vi "Initialize.vi"(8 "Error in (no error)":errorcluster, 9 "Reset":bool=TRUE caption="Reset (T)", 10 "ID Query":bool=TRUE caption="ID Query (T)", 11 "VISA resource":refnum<visa-resource-name>) -> (0 "Error out":errorcluster, 1 "THM1176 Description":string, 2 "THM1176":bool, 3 "Dup VISA resource":refnum<visa-resource-name>, 4 "Divisors":dbl[](array[numeric]) format="%#_8g", 5 "Ranges":string[](array[string]), 6 "Units":string[](array[string]))   [LabVIEW 2010]
doc: "Copyright (c) 2012 Metrolab Technology SA, Plan-les-Ouates, Geneva, Switzerland\nInitialize the THM1176 LabVIEW API."
panel:
  # "Initialize"
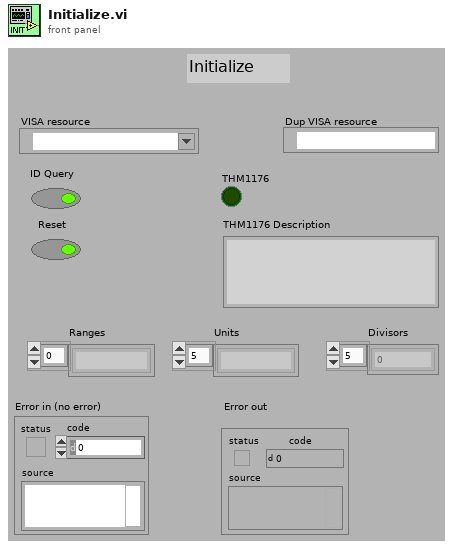
[diagram p1: front panel]
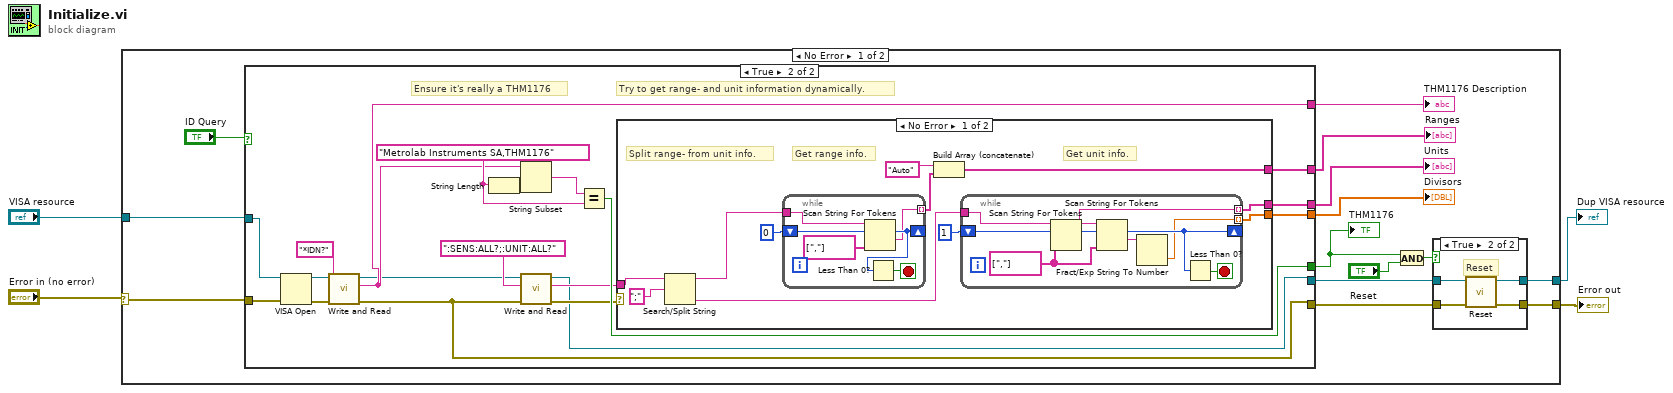
[diagram p0: block diagram]
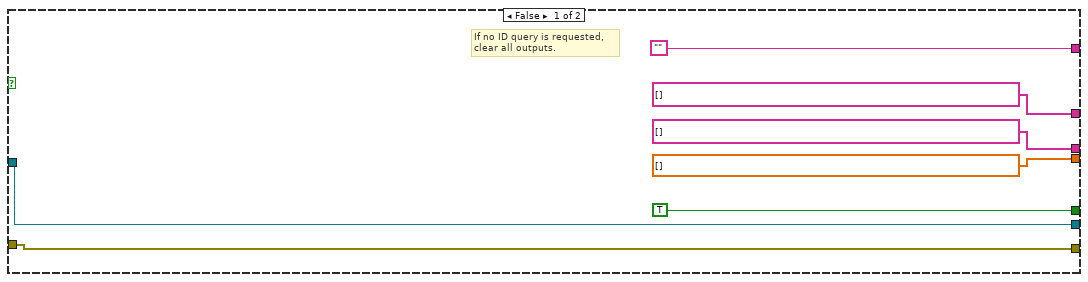
[diagram p2: hidden frame]
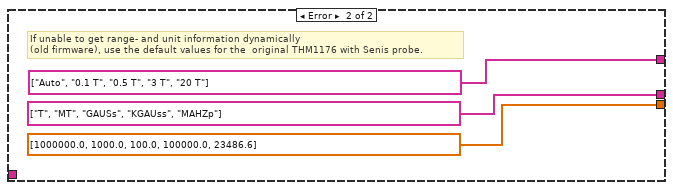
[diagram p3: hidden frame]
diagram:
  n1 = case shown="No Error" "Error in (no error)" {
    selector: "Error in (no error)" -> [w6 w82]
    tunnel: [w15 w81] -> w1
    tunnel: [w14 w82] -> w4
    tunnel: "VISA resource" -> [w5 w81]
    frame No Error {
      n2 = case shown="True" "ID Query" {
        tunnel: w6 -> [w25 w29]
        tunnel: [TRUE w36] -> w11
        tunnel: [w19 w31] -> w18
        tunnel: [w25 w33] -> w17
        tunnel: ["" ("response") w40] -> w13
        tunnel: [string[] [] w39] -> w9
        tunnel: [string[] [] w38] -> w8
        tunnel: [dbl[] [] w37] -> w7
        tunnel: w5 -> [w19 w27]
        frame False {
          # "If no ID query is requested,\nclear all outputs."
        }
        frame True {
          w42 = "Metrolab Instruments SA,THM1176"
          # "Try to get range- and unit information dynamically."
          # "Ensure it's really a THM1176"
          n3 = VISA Open(error in (no error)=w29, VISA resource name=w27) -> (VISA resource name=w26:refnum<visa-resource-name>, error out=w28:errorcluster)  [unwired: 3 in]
          n4 = call "Write and Read.vi"("Error in (no error)"=w28, "Command"="*IDN?" ("string to write"), "VISA resource"=w26) -> ("Error out"=w33:errorcluster, "Response"=w40:string, "Dup VISA resource"=w30:refnum<visa-resource-name>)  [unwired: 4 in, 2 out]
          n5 = String Length(string=w42) -> (length=w43:i32)
          n6 = String Subset(string=w40, length (rest)=w43) -> (substring=w41:string)  [unwired: 1 out]
          n7 = call "Write and Read.vi"("Error in (no error)"=w33, "Command"=":SENS:ALL?;:UNIT:ALL?", "VISA resource"=w30) -> ("Error out"=w34:errorcluster, "Response"=w32:string, "Dup VISA resource"=w31:refnum<visa-resource-name>)  [unwired: 4 in, 2 out]
          n8 = Equal?(x=w41, y=w42) -> (x = y?=w36:bool)
          n9 = case shown="No Error" w34 {
            tunnel: [w46 string[] ["Auto", "0.1 T", "0.5 T", "3 T", "20 T"]] -> w39
            tunnel: [w48 string[] ["T", "MT", "GAUSs", "KGAUss", "MAHZp"]] -> w38
            tunnel: [w47 dbl[] [1000000.0, 1000.0, 100.0, 100000.0, 23486.6]] -> w37
            tunnel: w32 -> [w54 _]
            frame No Error {
              # "Get unit info."
              # "Get range info."
              # "Split range- from unit info."
              n10 = Search/Split String(string=w54, search string/char (-)=";") -> (substring before match=w52:string, match + rest of string=w51:string)  [unwired: 2 out]
              n11 = while {
                shift-right: [w68] -> _
                shift-left: 0 ("offset past token") -> [w71]
                tunnel: w52 -> [w70]
                tunnel: [w66] -> w49 mode=indexing
                stop <- w67 stop-if-true
                n12 = Scan String For Tokens(6:string[] [","] ("delimiters (\\s,\\t,\\r,\\n)"), 8:w71, 9:w70) -> (1:w66:string, 2:w68:i32)  [unwired: 5 out]
                n13 = Less Than 0?(x=w68) -> (x < 0?=w67:bool)
              }
              n14 = Build Array (concatenate)("Auto", w49) -> (w46:string[])
              n15 = while {
                shift-right: [w60] -> _
                shift-left: 1 ("offset past token") -> [w65]
                tunnel: w51 -> [w64]
                tunnel: [w63] -> w48 mode=indexing
                tunnel: [w58] -> w47 mode=indexing
                stop <- w57 stop-if-true
                w61 = string[] [","] ("delimiters (\\s,\\t,\\r,\\n)")
                n16 = Scan String For Tokens(6:w61, 8:w65, 9:w64) -> (1:w63:string, 2:w62:i32, 3:w56:string)  [unwired: 4 out]
                n17 = Scan String For Tokens(6:w61, 8:w62, 9:w56) -> (1:w59:string, 2:w60:i32)  [unwired: 5 out]
                n18 = Fract/Exp String To Number(string=w59) -> (number=w58:dbl)  [unwired: 4 out]
                n19 = Less Than 0?(x=w60) -> (x < 0?=w57:bool)
              }
            }
            frame Error {
              # "If unable to get range- and unit information dynamically\n(old firmware), use the default values for the  original THM1176 with Senis probe."
            }
          }
        }
      }
      "THM1176" <- w11
      "THM1176 Description" <- w13
      "Ranges" <- w9
      "Units" <- w8
      "Divisors" <- w7
      n20 = And(x=w11, y="Reset") -> (x .and. y?=w12:bool)
      n21 = case shown="True" w12 {
        tunnel: w17 -> [w75 w80]
        tunnel: [w75 w79] -> w14
        tunnel: w18 -> [w76 w77]
        tunnel: [w76 w78] -> w15
        frame False {
        }
        frame True {
          # "Reset"
          n22 = call "Reset.vi"("Error in (no error)"=w80, "VISA resource"=w77) -> ("Error out"=w79:errorcluster, "Dup VISA resource"=w78:refnum<visa-resource-name>)  [unwired: 8 in]
        }
      }
    }
    frame Error {
    }
  }
  "Error out" <- w4
  "Dup VISA resource" <- w1
